vi "Write GoToNearBallPlacementSkill.vi"(8 "error in (no error)":errorcluster, 10 "GoToNearBallPlacementSkill":refnum<class "GoToNearBallPlacementSkill.lvclass">, 11 "Skillbook in":refnum<class "Skillbook.lvclass">) -> (0 "error out":errorcluster, 3 "Skillbook out":refnum<class "Skillbook.lvclass">)   [LabVIEW 2020, in "Skillbook.lvclass"]
uses:
  Skillbook.lvclass
  GoToNearBallPlacementSkill_class/GoToNearBallPlacementSkill.lvclass
  Skillbook.lvclass/Skillbook.ctl
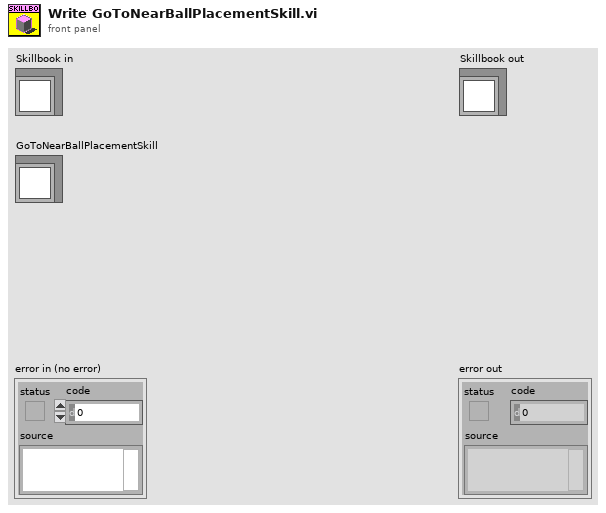
[diagram p1: front panel]
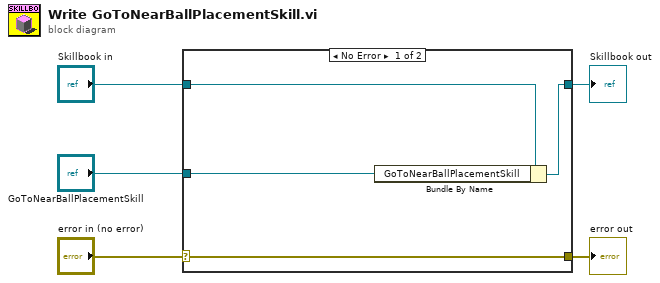
[diagram p0: block diagram]
diagram:
  n1 = case shown="No Error" "error in (no error)" {
    selector: "error in (no error)" -> [w9 w10]
    tunnel: [w9 w10] -> w4
    tunnel: [w7 w11] -> w2
    tunnel: "Skillbook in" -> [w8 w11]
    tunnel: "GoToNearBallPlacementSkill" -> [w6 _]
    frame No Error {
      n2 = Bundle By Name(cluster=w8, "GoToNearBallPlacementSkill"=w6) -> (w7:refnum<class "Skillbook.lvclass">)
    }
    frame Error {
    }
  }
  "error out" <- w4
  "Skillbook out" <- w2
